vi "4-dist.vi"(0 "err in 2":errorcluster caption="err in", 1 "p_LBin":T1) -> (2 "err in":errorcluster caption="err out", 3 "F":dbl[](array[numeric]), 4 "f":dbl[](array[numeric]), 5 "xk":i32[](array[numeric]))   [LabVIEW 2010, in "lv_02.lvlib"]
uses:
  lv_02.lvlib
  p_5E4_LBin.ctl
  4-k-dist.vi
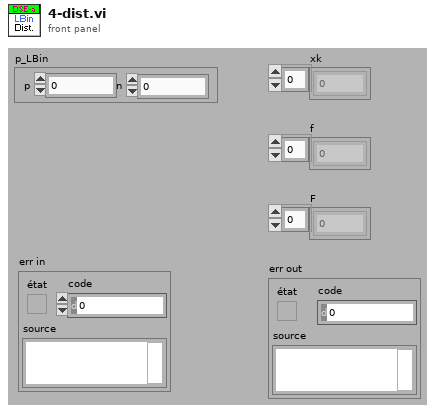
[diagram p1: front panel]
types:
  T1 = typedef "lv_02.lvlib/p_5E4_LBin.ctl" = cluster{"p":dbl, "n":i16}
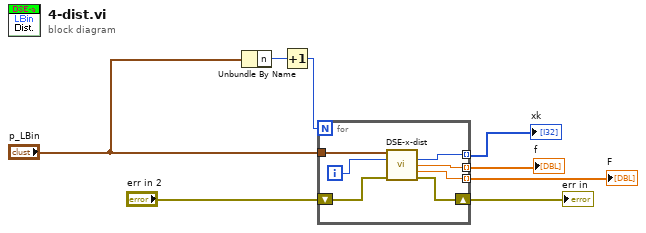
[diagram p0: block diagram]
diagram:
  n1 = Unbundle By Name("p_LBin") -> ("n"=w6:i16)
  n2 = Increment(x=w6) -> (x+1=w3:i16)
  n3 = for {
    N: w3 -> [_]
    tunnel: [w13] -> w1 mode=indexing
    tunnel: [w12] -> w4 mode=indexing
    tunnel: [w11] -> w2 mode=indexing
    tunnel: "p_LBin" -> [w15]
    shift-right: [w10] -> w8
    shift-left: "err in 2" -> [w9]
    i -> [w14]
    n4 = call-poly "DSE-x-dist.vi"("p_LBin"=w15, "X=k"=w14, "error in (no error)"=w9) -> ("X=k"=w13:i32, "f(X=k)"=w12:dbl, "Fr(X=k)"=w11:dbl, "error out"=w10:errorcluster)  [unwired: 8 in, 1 out]
  }
  "err in" <- w8
  "f" <- w4
  "F" <- w2
  "xk" <- w1
